vi "Custom Format Start Index.vi"() -> (3 "Start ID":u32=164)   [LabVIEW 2019, in "Open Xml.lvlib"]
uses:
  Open Xml.lvlib
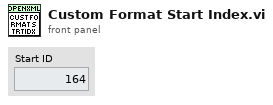
[diagram p1: front panel]
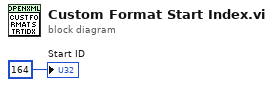
[diagram p0: block diagram]
diagram:
  "Start ID" <- u32 164
